vi "Get Crafting Stations.vi"(8 "error in (no error)":errorcluster, 11 "Chemicals in":refnum<class "Chemicals.lvclass">) -> (0 "error out":errorcluster, 2 "Stations":T1[](array[typedef]), 3 "Chemicals out":refnum<class "Chemicals.lvclass">)   [LabVIEW 2020, in "Chemicals.lvclass"]
uses:
  Chemicals.lvclass
  Item/Craft Station.ctl
  Workstation/Workstation.lvclass
  Item/Item.lvclass
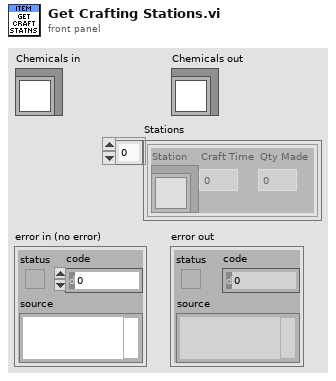
[diagram p1: front panel]
types:
  T1 = typedef "Item.lvclass/Craft Station.ctl" = cluster{"Station":refnum<class "Workstation.lvclass">, "Craft Time":dbl, "Qty Made":dbl}
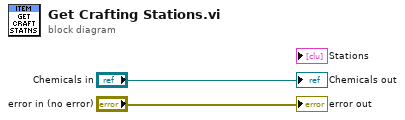
[diagram p0: block diagram]
diagram:
  "error out" <- "error in (no error)"
  "Chemicals out" <- "Chemicals in"
